vi "Untitled 1.vi"() -> ()   [LabVIEW 2015]
uses:
  <vilib>/Utility/SystemLogging/NI_SystemLogging.lvlib
panel:
  out "data":string
  out "error out":errorcluster
  in  "data name":string
  in  "type":string
  in  "error in":errorcluster
  in  "Tab Control":T1(tab)
  in  "itterations":i32
  out "Output Array 1":dbl[](array[numeric])
  in  "default value 2":dbl
  in  "array  size":i32
  out "size(s)":i32
  out "size(s) 2":i32
  in  "default value":dbl
  in  "array size":i32
  out "output Array 2":dbl[](array[numeric])
  out "Numeric":i32
  out "size(s) 3":i32
  out "size(s) 4":i32
  out "max value":dbl
  out "max index(es)":i32
  out "min value":dbl
  out "min index(es)":i32
  out "output array":dbl[](array[numeric])
  in  "index":i32
  out "appended array":dbl[][](array[numeric])
  in  "element":dbl
  in  "dimension size":i32
  in  "element 2":dbl
  in  "dimension size 2":i32
  out "concatenate array 2":dbl[](array[numeric])
  in  "element 3":dbl
  in  "dimension size 3":i32
  in  "element 4":dbl
  in  "dimension size 4":i32
  in  "element 5":dbl
  in  "dimension size 5":i32
  in  "element 6":dbl
  in  "dimension size 6":i32
  in  "index 2":i32
  in  "length":i32
  in  "index 3":i32
  in  "length 2":i32
  out "subarray":dbl[][](array[numeric])
  out "Array":dbl[][](array[numeric])
  in  "element 7":dbl
  in  "dimension size 7":i32
  in  "element 8":dbl
  in  "dimension size 8":i32
  in  "element 9":dbl
  in  "dimension size 9":i32
  in  "array":dbl[](array[numeric])
  in  "2D array":i32
  out "output array 2":dbl[][][](array[numeric])
  in  "1D array":i32
  in  "elements":i32
  out "*C Thermometer o/p":dbl(slide) scale=0.0..100.0
  in  "*F Thermometer":dbl(slide) scale=0.0..100.0
  out "*F Thermometer o/p":dbl(slide) scale=0.0..100.0
  in  "*C Thermometer":dbl(slide) scale=0.0..100.0
  in  "stop":bool
  in  "Array 2":string[][](array[string])
  out "length 3":i32[][](array[numeric])
  out "result string":string
  in  "UTC format":bool
  in  "time stamp":timestamp
  in  "time format string (%c)":string
  in  "dimension size 10":i32
  out "element 10":string
  in  "dimension size 11":i32
  in  "dimension size 12":i32
  in  "dimension size 13":i32
  in  "dimension size 14":i32
  out "array of clusters":cluster{string[]}[](array[cluster])
  in  "Cluster":T2
  out "Numeric 2":dbl
  out "Boolean":bool
  out "String":string
  out "Numeric 3":dbl
  in  "millisecond multiple":u32
  out "millisecond timer value":u32
  in  "milliseconds to wait":u32
  out "millisecond timer value 2":u32
  in  "milliseconds to wait 2":u32
  in  "y":dbl
  in  "x":dbl
  out "x = y?":bool
  out "millisecond timer value 3":u32
  out "millisecond timer value 4":u32
  out "total time taken":u32
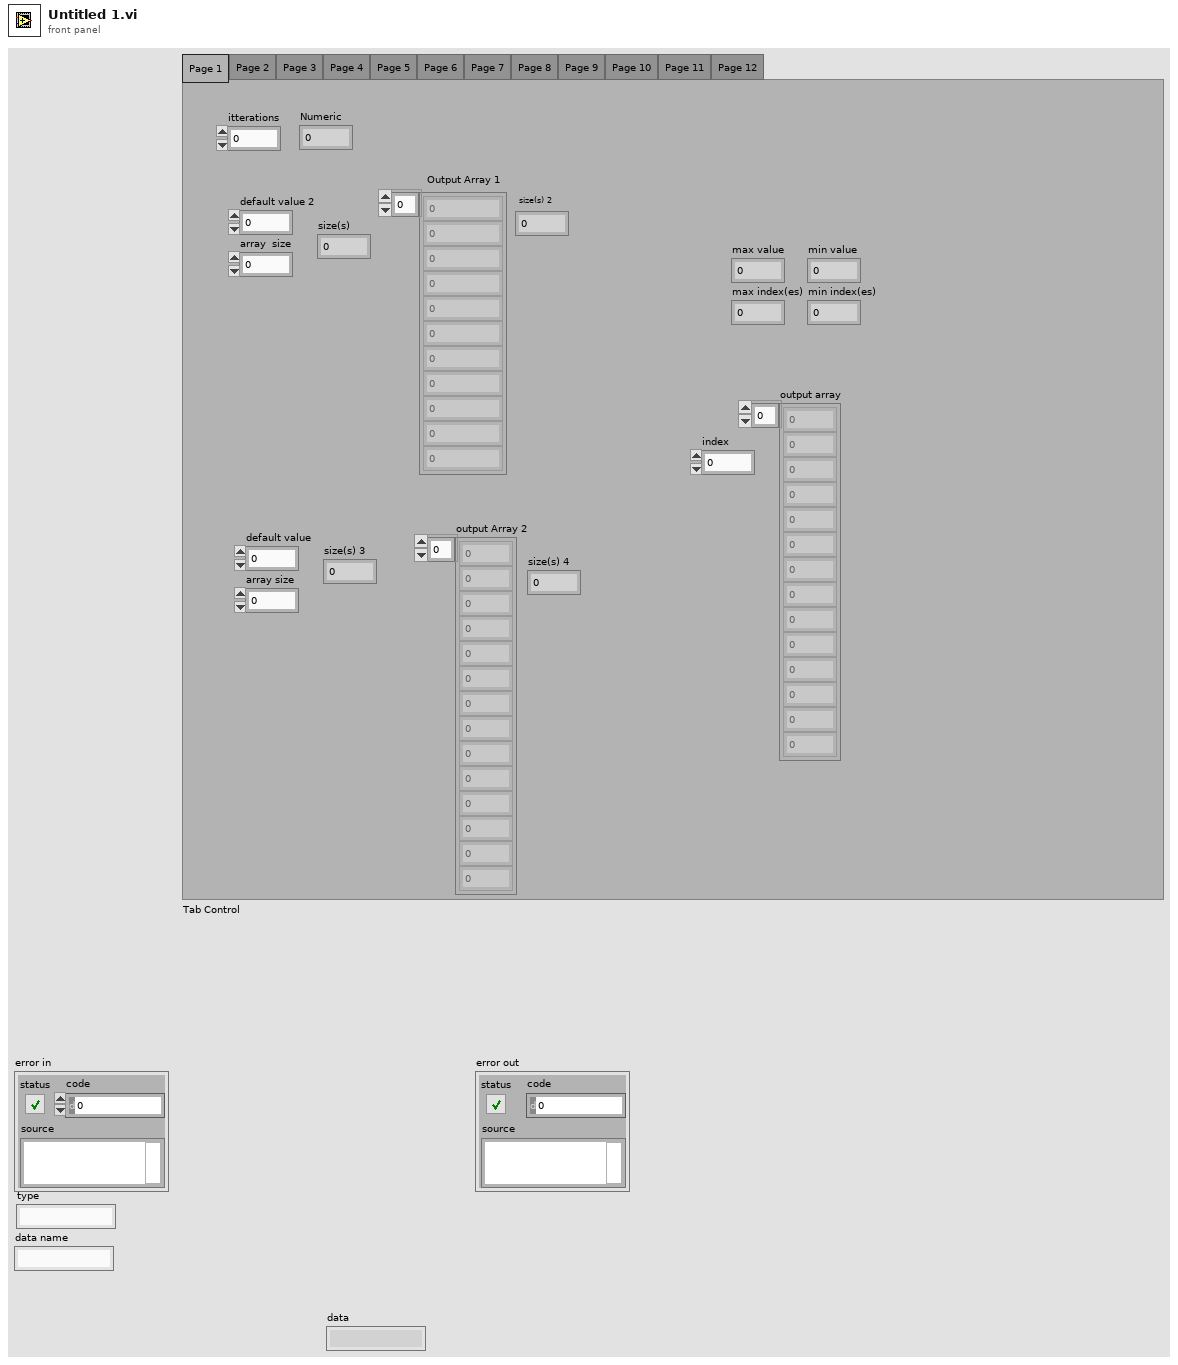
[diagram p1: front panel]
types:
  T1 = enum32{"Page 1", "Page 2", "Page 3", "Page 4", "Page 5", "Page 6", "Page 7", "Page 8", "Page 9", "Page 10", "Page 11", "Page 12"}
  T2 = cluster{"Numeric":dbl, "Boolean":bool, "Boolean 2":bool, "String":string}
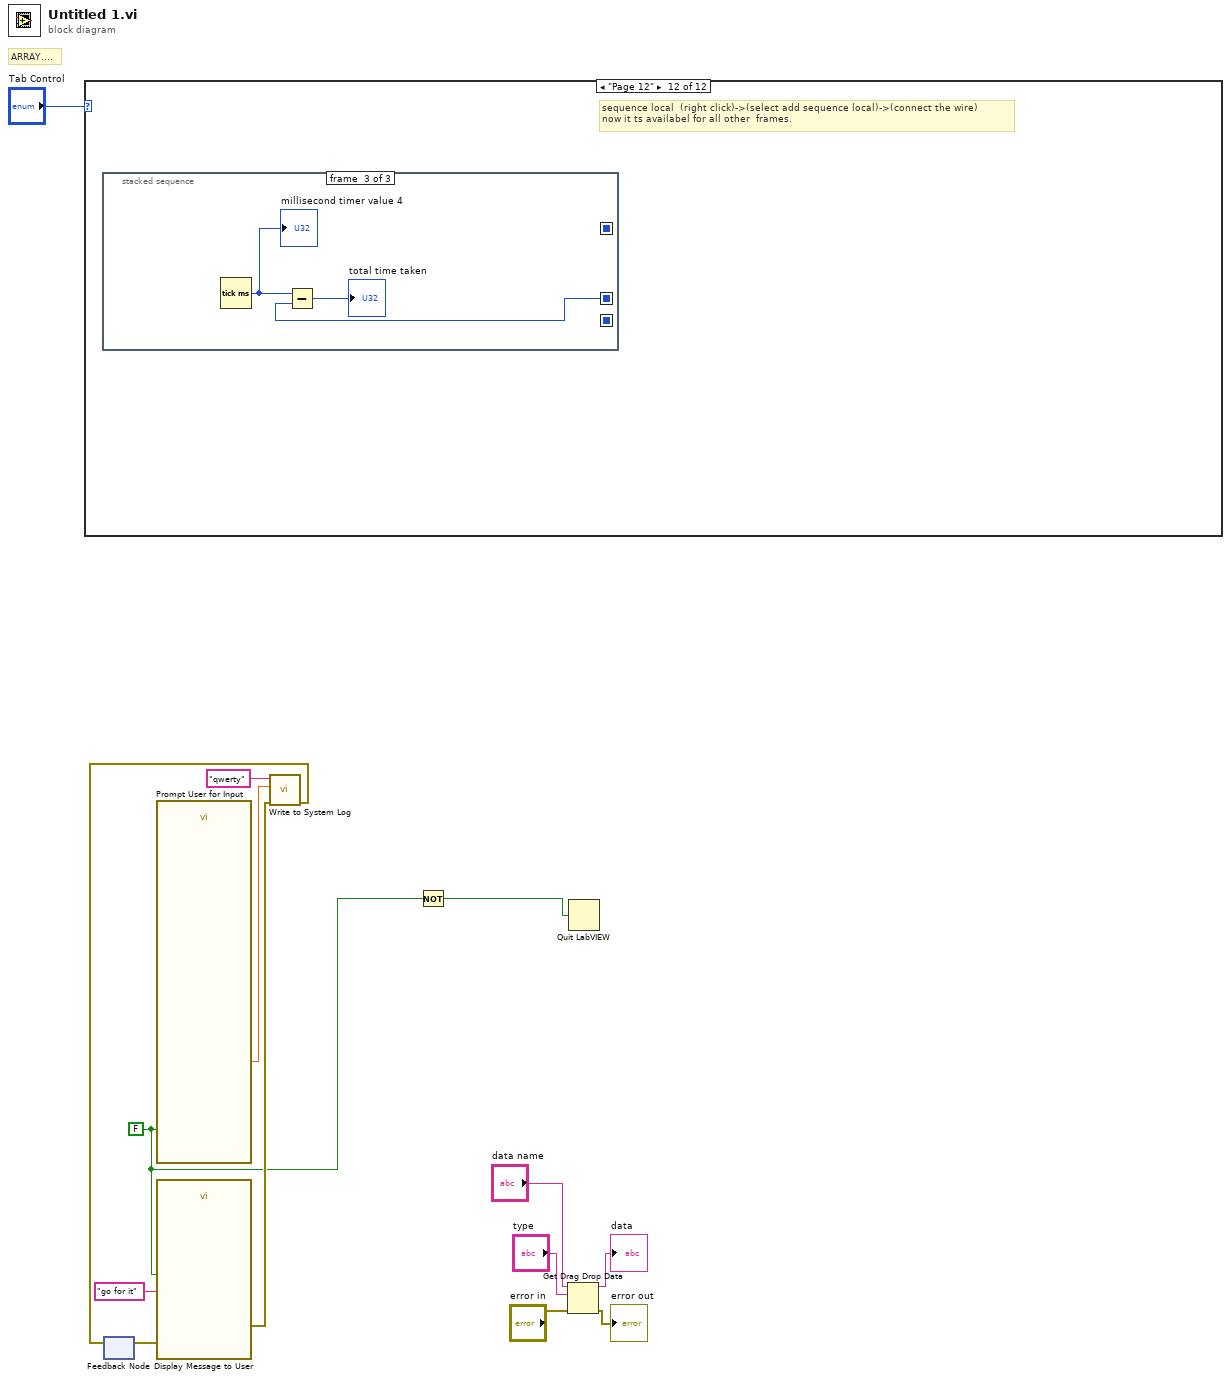
[diagram p0: block diagram]
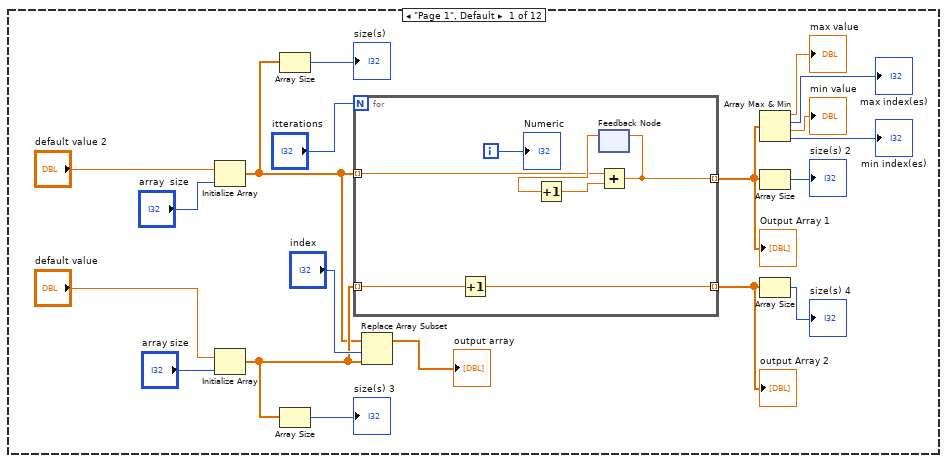
[diagram p2: hidden frame]
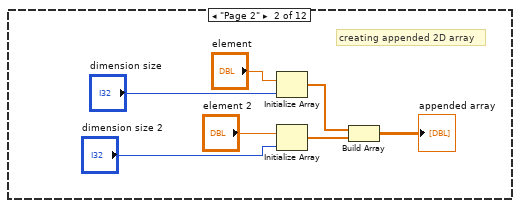
[diagram p3: hidden frame]
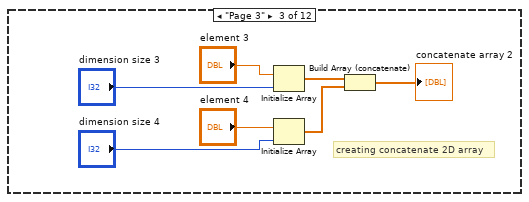
[diagram p4: hidden frame]
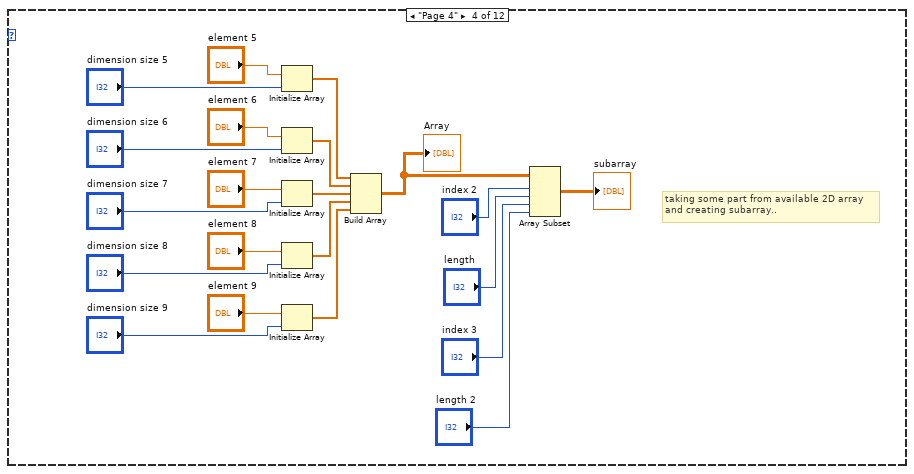
[diagram p5: hidden frame]
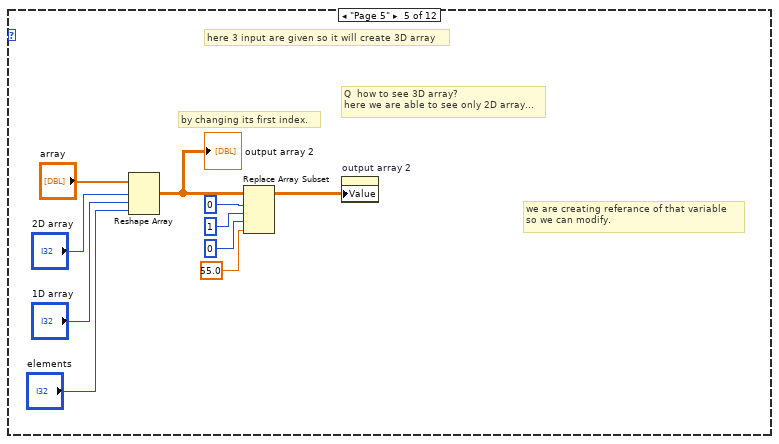
[diagram p6: hidden frame]
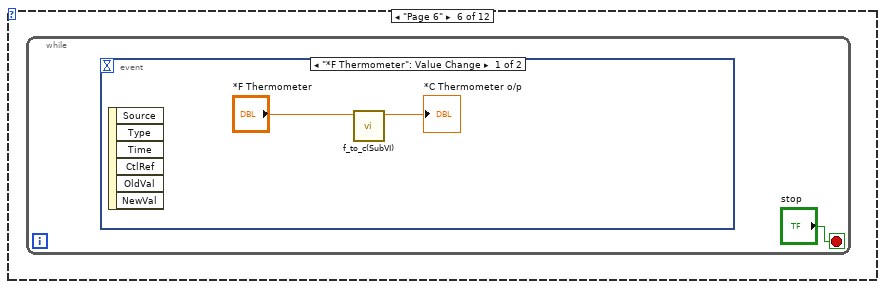
[diagram p7: hidden frame]
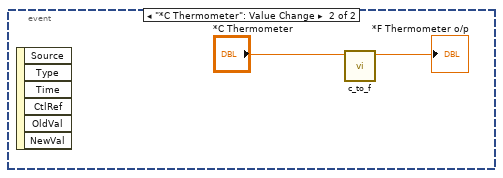
[diagram p8: hidden frame]
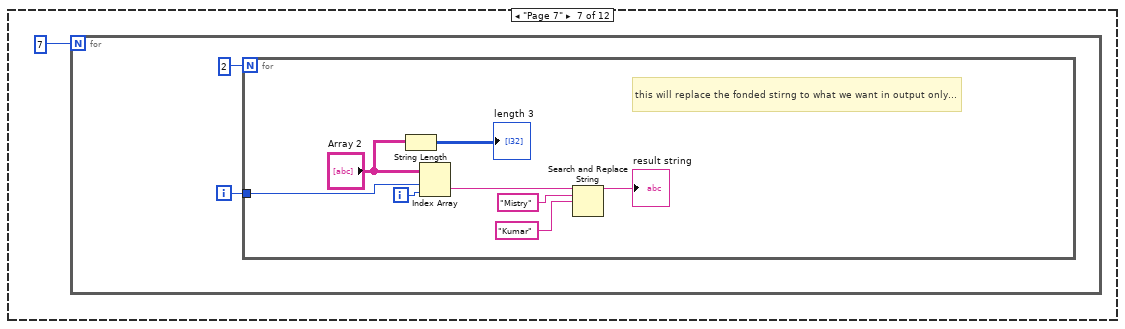
[diagram p9: hidden frame]
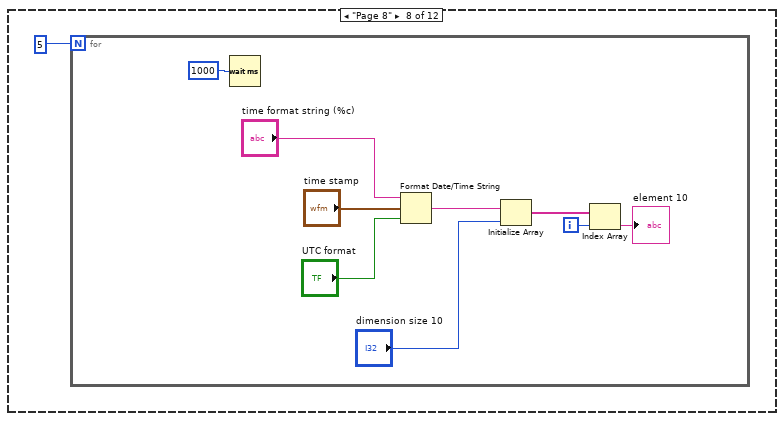
[diagram p10: hidden frame]
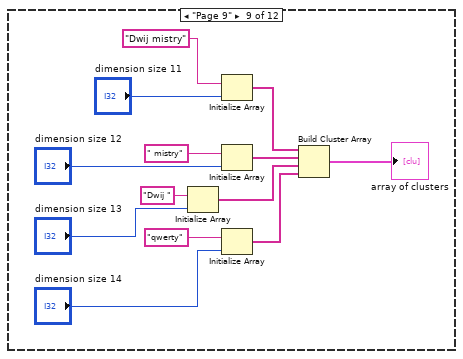
[diagram p11: hidden frame]
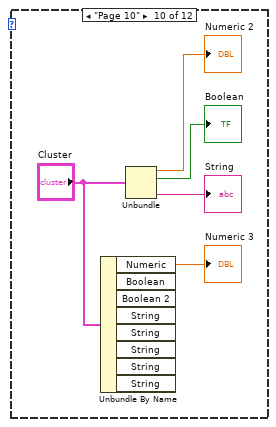
[diagram p12: hidden frame]
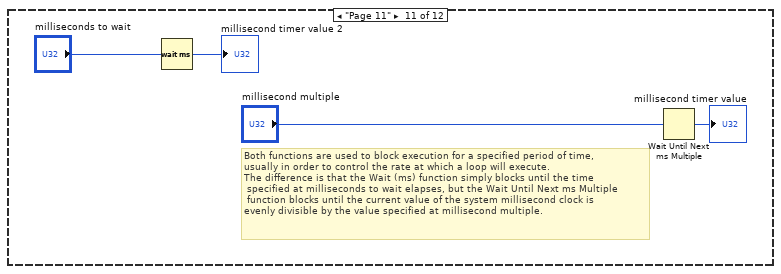
[diagram p13: hidden frame]
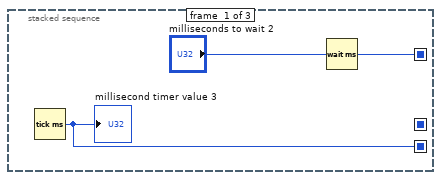
[diagram p14: hidden frame]
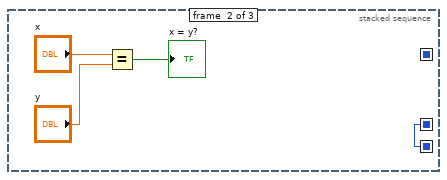
[diagram p15: hidden frame]
diagram:
  w1 = FALSE ("Enable")
  # "ARRAY...."
  n1 = case shown="\"Page 12\"" "Tab Control" {
    frame "Page 1", Default {
      n2 = Initialize Array("default value 2", "array  size") -> (w30:dbl[])
      n3 = Initialize Array("default value", "array size") -> (w31:dbl[])
      n4 = Array Size(array=w30) -> (size(s)=→"size(s)":i32)
      n5 = Array Size(array=w31) -> (size(s)=→"size(s) 3":i32)
      n6 = for {
        N: "itterations" -> [_]
        tunnel: w31 -> [w40] mode=indexing
        tunnel: [w39] -> w23 mode=indexing
        tunnel: w30 -> [w35] mode=indexing
        tunnel: [w34] -> w25 mode=indexing
        i -> [w38]
        n7 = Increment(x=w40) -> (x+1=w39:dbl)
        n8 = feedback #1() -> (w36:dbl)  [unwired: 1 in]
        n9 = Increment(x=w36) -> (x+1=w37:dbl)
        n10 = Add(x=w35, y=w37) -> (x+y=w34:dbl)
        n11 = feedback-in #1(w34) -> ()
        "Numeric" <- w38
      }
      "Output Array 1" <- w25
      "output Array 2" <- w23
      n12 = Replace Array Subset(array=w30, new element=w31, index="index") -> (→"output array":dbl[])
      n13 = Array Max & Min(array=w25) -> (max value=→"max value":dbl, max index (indices)=→"max index(es)":i32, min value=→"min value":dbl, min index (indices)=→"min index(es)":i32)
      n14 = Array Size(array=w25) -> (size(s)=→"size(s) 2":i32)
      n15 = Array Size(array=w23) -> (size(s)=→"size(s) 4":i32)
    }
    frame "Page 2" {
      # "creating appended 2D array"
      n16 = Initialize Array("element", "dimension size") -> (w44:dbl[])
      n17 = Initialize Array("element 2", "dimension size 2") -> (w45:dbl[])
      n18 = Build Array(w44, w45) -> (→"appended array":dbl[][])
    }
    frame "Page 3" {
      # "creating concatenate 2D array"
      n19 = Initialize Array("element 3", "dimension size 3") -> (w51:dbl[])
      n20 = Initialize Array("element 4", "dimension size 4") -> (w52:dbl[])
      n21 = Build Array (concatenate)(w51, w52) -> (→"concatenate array 2":dbl[])
    }
    frame "Page 4" {
      # "taking some part from available 2D array\nand creating subarray.."
      n22 = Initialize Array("element 5", "dimension size 5") -> (w57:dbl[])
      n23 = Initialize Array("element 6", "dimension size 6") -> (w60:dbl[])
      n24 = Initialize Array("element 7", "dimension size 7") -> (w71:dbl[])
      n25 = Initialize Array("element 8", "dimension size 8") -> (w72:dbl[])
      n26 = Initialize Array("element 9", "dimension size 9") -> (w75:dbl[])
      n27 = Build Array(w57, w60, w71, w72, w75) -> (w66:dbl[][])
      "Array" <- w66
      n28 = Array Subset(array=w66, index (row)="index 2", length (row)="length", index (col)="index 3", length (col)="length 2") -> (→"subarray":dbl[][])
    }
    frame "Page 5" {
      # "by changing its first index."
      # "we are creating referance of that variable \nso we can modify."
      # "Q  how to see 3D array?\nhere we are able to see only 2D array..."
      # "here 3 input are given so it will create 3D array"
      n29 = Reshape Array("array", "2D array", "1D array", "elements") -> (w81:dbl[][][])
      "output array 2" <- w81
      n30 = Replace Array Subset(array=w81, new element=55.0 ("new element/subarray"), index (dim 0)=0 ("index (page)"), index (dim 1)=1 ("disabled index (row)"), index (dim 2)=0 ("disabled index (col)")) -> (w76:dbl[][][])
      n31 = property on="output array 2" class="Arr (strict)"("Value"=w76) -> ()  [unwired: 2 in, 2 out]
    }
    frame "Page 6" {
      n32 = while {
        stop <- "stop" stop-if-true
        n33 = event shown="[0] \"*F Thermometer\": Value Change" {
          selector: _ -> [_ _]
          dyn-events: _ -> [_ _]
          timeout: _ -> [_ _]
          event "*F Thermometer": Value Change {
            n34 = event-data() -> ()  [unwired: 1 in, 6 out]
            n35 = call "f_to_c(SubVI).vi"("*F Thermometer"="*F Thermometer") -> ("Numeric"=→"*C Thermometer o/p":dbl)  [unwired: 10 in]
          }
          event "*C Thermometer": Value Change {
            n36 = event-data() -> ()  [unwired: 1 in, 6 out]
            n37 = call "c_to_f.vi"("*C Thermometer"="*C Thermometer") -> ("Numeric"=→"*F Thermometer o/p":dbl)  [unwired: 10 in]
          }
        }
      }
    }
    frame "Page 7" {
      n38 = for {
        N: 7 -> [_]
        i -> [w93]
        n39 = for {
          N: 2 -> [_]
          tunnel: w93 -> [w99]
          i -> [w98]
          # "this will replace the fonded stirng to what we want in output only..."
          n40 = String Length(string="Array 2") -> (length=→"length 3":i32[][])
          n41 = Index Array(array="Array 2", index (row)=w99, index (col)=w98) -> (element=w97:string)
          n42 = Search and Replace String(input string=w97, search string="Mistry", replace string="Kumar" ("replace string (\"\")")) -> (result string=→"result string":string)  [unwired: 5 in, 3 out]
        }
      }
    }
    frame "Page 8" {
      n43 = for {
        N: 5 -> [_]
        i -> [w105]
        n44 = Wait (ms)(milliseconds to wait=u32 1000) -> ()  [unwired: 1 out]
        n45 = Format Date/Time String(time format string (%c)="time format string (%c)", seconds (now)="time stamp", UTC format="UTC format") -> (date/time string=w104:string)
        n46 = Initialize Array(w104, "dimension size 10") -> (w106:string[])
        n47 = Index Array(array=w106, index=w105) -> (element=→"element 10":string)
      }
    }
    frame "Page 9" {
      n48 = Initialize Array("Dwij ", "dimension size 13") -> (w118:string[])
      n49 = Initialize Array("Dwij mistry", "dimension size 11") -> (w122:string[])
      n50 = Initialize Array(" mistry", "dimension size 12") -> (w117:string[])
      n51 = Initialize Array("qwerty", "dimension size 14") -> (w121:string[])
      n52 = Build Cluster Array(w122, w117, w118, w121) -> (→"array of clusters":cluster{string[]}[])
    }
    frame "Page 10" {
      n53 = Unbundle By Name("Cluster") -> ("Numeric"=→"Numeric 3":dbl)  [unwired: 7 out]
      n54 = Unbundle("Cluster") -> ("Numeric"=→"Numeric 2":dbl, "Boolean"=→"Boolean":bool, "String"=→"String":string)  [unwired: 1 out]
    }
    frame "Page 11" {
      # "Both functions are used to block execution for a specified period of time, \nusually in order to control the rate at which a loop will execute. \nThe difference is that the Wait (ms) function simply blocks until the time\n specified at milliseconds to wait elapses, but the Wait Until Next ms Multiple\n function blocks until the current value of the system millisecond clock is \nevenly divisible by the value specified at millisecond multiple."
      n55 = Wait (ms)(milliseconds to wait="milliseconds to wait") -> (millisecond timer value=→"millisecond timer value 2":u32)
      n56 = Wait Until Next ms Multiple(millisecond multiple="millisecond multiple") -> (millisecond timer value=→"millisecond timer value":u32)
    }
    frame "Page 12" {
      # "sequence local  (right click)->(select add sequence local)->(connect the wire) \nnow it ts availabel for all other  frames."
      n57 = stacked-sequence {
        seq-local: [w135 _ _] -> [_ w137 _]
        seq-local: [_ w137 _] -> [_ _ w142]
        seq-local: [w134 _ _] -> [_ _ _]
        frame #0 {
          n58 = Tick Count (ms)() -> (millisecond timer value=w135:u32)
          "millisecond timer value 3" <- w135
          n59 = Wait (ms)(milliseconds to wait="milliseconds to wait 2") -> (millisecond timer value=w134:u32)
        }
        frame #1 {
          n60 = Equal?(x="x", y="y") -> (x = y?=→"x = y?":bool)
        }
        frame #2 {
          n61 = Tick Count (ms)() -> (millisecond timer value=w143:u32)
          "millisecond timer value 4" <- w143
          n62 = Subtract(x=w143, y=w142) -> (x-y=→"total time taken":u32)
        }
      }
    }
  }
  n63 = feedback #2() -> (w8:errorcluster)  [unwired: 1 in]
  n64 = call "Prompt User for Input"("Enable"=w1) -> ("g"=w11:dbl)  [unwired: 8 in, 10 out]
  n65 = call "Display Message to User"("error in (no error)"=w8, "Enable"=w1, "Message"="go for it") -> ("error out"=w10:errorcluster)  [unwired: 7 in, 1 out]
  n66 = call <vilib>:"Write to System Log.vi"("error in (no error)"=w10, "severity"=w11, "message"="qwerty") -> ("error out"=w9:errorcluster)  [unwired: 8 in]
  n67 = feedback-in #2(w9) -> ()
  n68 = Not(x=w1) -> (.not. x?=w2:bool)
  n69 = Get Drag Drop Data(6:"error in", 8:"type", 9:"data name") -> (0:→"error out":errorcluster, 3:→"data":string)
  n70 = Quit LabVIEW(quit? (T)=w2) -> ()
